vi "信号监控.vi"() -> ()   [LabVIEW 2015]
uses:
  Global control/global-1.vi
  Global control/global-opc.vi
  <userlib>/QMH/Message Queue/Support/Enqueue Message (Single).vi
  Global control/global-2.vi
  <userlib>/QMH/User Event - Stop/User Event - Stop.lvlib
  <userlib>/QMH/Message Queue/Message Queue.lvlib
panel:
  in  "切换界面":bool
  in  "HostThread":variant
  in  "Exit":bool
  in  "选项卡控件":enum32{"继保信号", "管理机信号", "柜体信号"}(tab)
  in  "直流屏-遥测":bool
  in  "直流屏-遥信":bool
  in  "继保选项卡":enum32{"继遥信", "继遥测", "继遥控"}(tab)
  out "继保遥信":T1
  out "继保遥测":T2
  in  "继保遥控":cluster{"断路器分闸":bool, "断路器合闸":bool}
  in  "管理机选项卡":enum32{"管遥信", "管遥测"}(tab)
  out "管理机遥信":T3
  out "管理机遥测":T4 {"主机交流输入电压C相" format="%1.1f"; "主机交流输入电压B相" format="%1.1f"; "主机交流输入电压A相" format="%1.1f"; "母线对地交流电压" format="%1.1f"; "母线负对地电阻" format="%1.1f"; "母线正对地电阻" format="%1.1f"; "母线负对地电压" format="%1.1f"; "母线正对地电压" format="%1.1f"; "负载电流" format="%1.1f"; "母线电压" format="%1.1f"; "电池组温度" format="%1.1f"; "电池组电流" format="%1.1f"; "电池组电压" format="%1.1f"}
  in  "PLC选项卡":T5(tab)
  out "PLC-整流器柜遥测":T6 {"10KV电压输入" format="%1.1f"; "直流1500V电压输出" format="%1.1f"; "直流电流输出" format="%1.1f"}
  in  "PLC-整流器柜遥控":cluster{"模拟中压合闸控制":bool}
  out "PLC-整流器柜遥信":T7
  in  "PLC-直流进线柜遥控":T8
  out "PLC-直流进线柜遥信":T9
  out "PLC-直流馈线柜遥测":cluster{"DC1500V电压输出":dbl} {"DC1500V电压输出" format="%1.1f"}
  in  "PLC-直流馈线柜遥控":T10
  out "PLC-直流馈线柜遥信":T11
  in  "PLC-负极柜遥信遥控":T12
  out "PLC-负极柜遥信":T13
  in  "PLC-接触网隔离开关柜遥控":cluster{"刀开关合闸控制":bool, "刀开关分闸控制":bool}
  out "PLC-接触网隔离开关柜遥信":T14
  # "继保监控"
  # "遥信"
  # "软压板"
  # "开入"
  # "遥测"
  # "遥控"
  # "管理机监控"
  # "遥信"
  # "遥测"
  # "柜体监控"
  # "遥测"
  # "遥控"
  # "遥信"
  # "遥控"
  # "遥信"
  # "遥测"
  # "遥控"
  # "遥信"
  # "遥控"
  # "遥信"
  # "遥控"
  # "遥信"
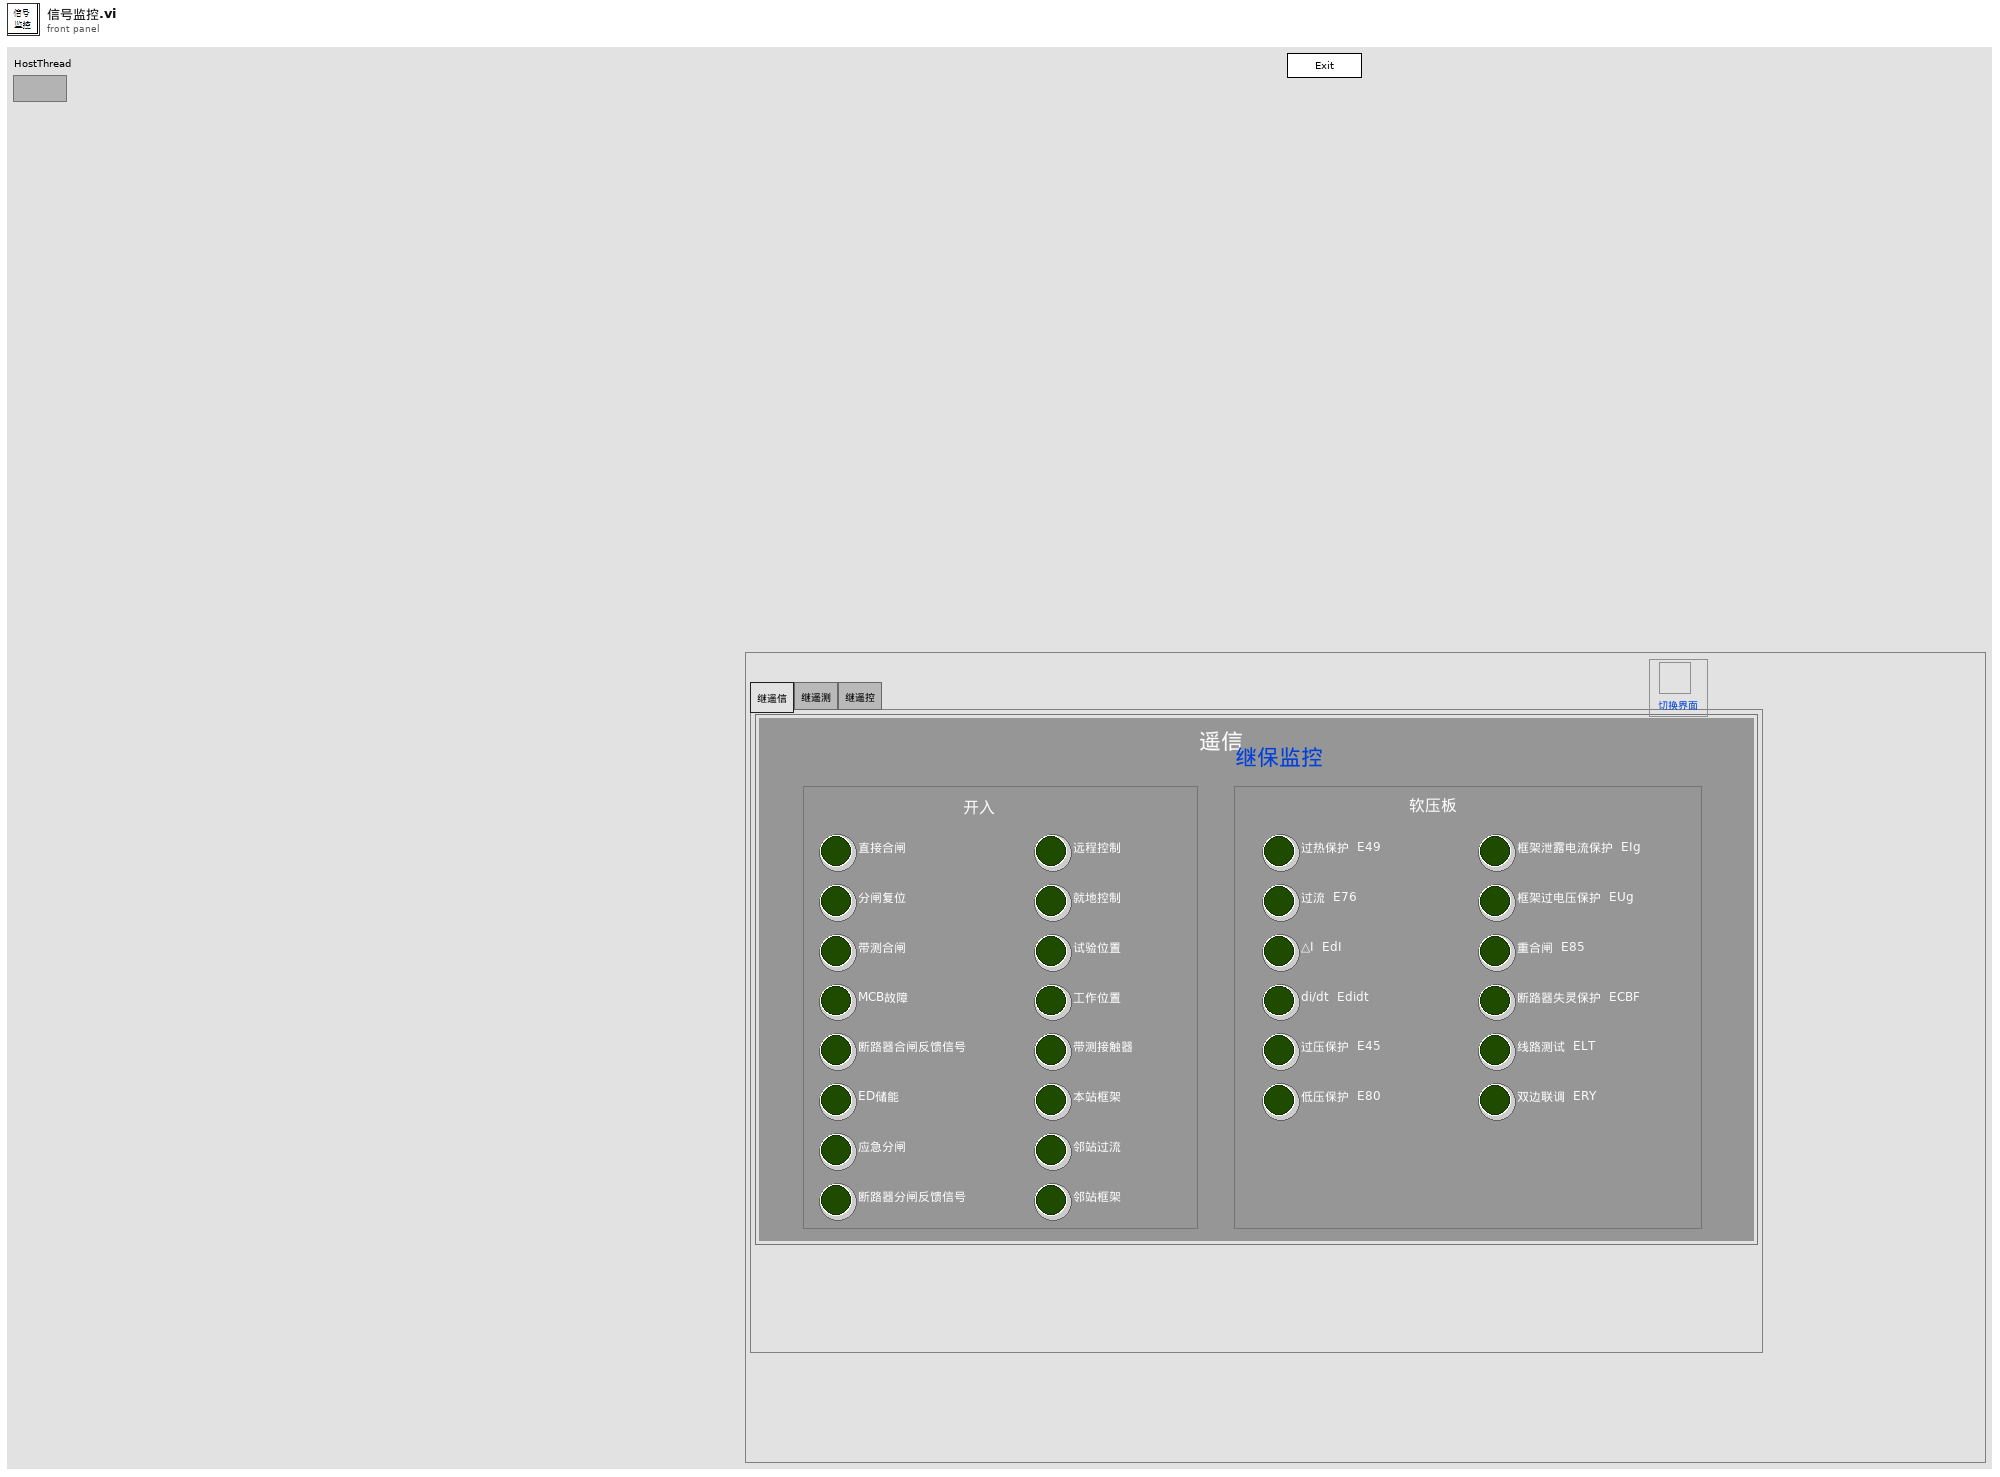
[diagram p1: front panel]
types:
  T1 = cluster{"直接合闸":bool, "分闸复位":bool, "带测合闸":bool, "MCB故障":bool, "断路器合闸反馈信号":bool, "ED储能":bool, "应急分闸":bool, "断路器分闸反馈信号":bool, "远程控制":bool, "就地控制":bool, "试验位置":bool, "工作位置":bool, "带测接触器":bool, "本站框架":bool, "邻站过流":bool, "邻站框架":bool, "过热保护  E49":bool, "过流  E76":bool, "△I  EdI":bool, "di/dt  Edidt":bool, "过压保护  E45":bool, "低压保护  E80":bool, "框架泄露电流保护  EIg":bool, "框架过电压保护  EUg":bool, "重合闸  E85":bool, "断路器失灵保护  ECBF":bool, "线路测试  ELT":bool, "双边联调  ERY":bool}
  T2 = cluster{"电流（I）":u32, "电压（U）":u32, "功率（W）":u32, "框架电流（Ig）":u32, "框架电压（UgV）":u32, "过热余量(Tem)":u32, "电流上升率（didt）":u32, "线路测试状态（LTState）":u32, "重合闸状态（RCLState）":u32}
  T3 = cluster{"母线过压":bool, "母线欠压":bool, "母线绝缘异常":bool, "母线绝缘预警":bool, "母线绝缘压差故障":bool, "母线交流串入故障":bool, "电池组过压":bool, "电池组欠压":bool, "电池组过温":bool, "单体电池故障":bool, "Host交流故障":bool, "Host交流缺相":bool, "Host交流失电":bool, "01#JLCL交流故障":bool, "01#JLCL交流缺相":bool, "01#JLCL交流失电":bool, "02#JLCL交流故障":bool, "02#JLCL交流缺相":bool, "02#JLCL交流失电":bool, "01#电源模块故障":bool, "02#电源模块故障":bool, "03#电源模块故障":bool, "01#模块通信故障":bool, "02#模块通信故障":bool, "03#模块通信故障":bool, "控母输出1#告警":bool, "控母输出2#告警":bool, "控母输出3#告警":bool, "控母输出4#告警":bool, "控母输出5#告警":bool, "控母输出6#告警":bool, "合母输出1#告警":bool, "合母输出2#告警":bool, "合母输出3#告警":bool, "合母输出4#告警":bool, "合母输出5#告警":bool, "合母输出6#告警":bool, "交流输入I告警":bool, "交流输入II告警":bool}
  T4 = cluster{"电池组电压":dbl, "电池组电流":dbl, "电池组温度":dbl, "母线电压":dbl, "负载电流":dbl, "母线正对地电压":dbl, "母线负对地电压":dbl, "母线正对地电阻":dbl, "母线负对地电阻":dbl, "母线对地交流电压":dbl, "主机交流输入电压A相":dbl, "主机交流输入电压B相":dbl, "主机交流输入电压C相":dbl}
  T5 = enum32{"整流器柜", "直流进线柜", "直流馈线柜", "负极柜", "接触网隔离开关柜"}
  T6 = cluster{"直流电流输出":dbl, "直流1500V电压输出":dbl, "10KV电压输入":dbl}
  T7 = cluster{"正常运行":bool, "异常跳闸":bool, "远方":bool, "负极柜故障":bool, "正极柜故障":bool, "馈线柜故障":bool, "接触网隔离开关柜故障":bool, "整流柜跳闸":bool, "整流柜合闸":bool, "压敏快熔故障":bool, "整流柜故障":bool, "模拟中压合闸":bool, "本地":bool}
  T8 = cluster{"刀开关合闸控制":bool, "刀开关分闸控制":bool, "故障复位控制":bool}
  T9 = cluster{"正常运行":bool, "设备准备好":bool, "设备异常":bool, "刀开关合闸完成":bool, "刀开关分闸完成":bool, "刀开关合闸":bool, "刀开关分闸":bool, "复位":bool, "远方":bool, "本地":bool, "刀开关合闸进行中":bool, "刀开关分闸进行中":bool}
  T10 = cluster{"高断储能控制":bool, "旁路合闸控制":bool, "旁路分闸控制":bool, "断路器分闸":bool, "断路器合闸":bool}
  T11 = cluster{"正常运行":bool, "设备准备好":bool, "设备异常":bool, "高断合闸完成":bool, "高断分闸完成":bool, "旁路合闸":bool, "旁路分闸":bool, "继保故障信号":bool, "远方":bool, "本地":bool, "旁路合闸完成":bool, "允许高断合闸":bool}
  T12 = cluster{"模拟框架电流故障控制":bool, "模拟框架电压故障控制":bool, "模拟I段电压故障":bool, "模拟II段电压故障":bool, "故障复位控制":bool}
  T13 = cluster{"正常运行":bool, "设备准备好":bool, "设备异常":bool, "II段电压故障":bool, "MCB故障":bool, "刀开关合闸完成":bool, "复位":bool, "远方":bool, "本地":bool, "装置故障":bool, "刀开关合闸进行中":bool, "框架电流故障":bool, "I段电压故障":bool, "框架电压故障":bool, "刀开关分闸完成":bool}
  T14 = cluster{"正常运行":bool, "设备准备好":bool, "设备异常":bool, "刀开关合闸完成":bool, "刀开关分闸完成":bool, "接触轨有压":bool, "远方":bool, "本地":bool, "刀开关分闸进行中":bool, "刀开关合闸进行中":bool, "刀开关分闸":bool, "刀开关合闸":bool}
  T15 = cluster{"Controls":cluster{"Exit":refnum<vi>}, "Thread":cluster{"ThisQ":string, "ThisVI":refnum<vi>, "HostQ":string, "HostRef":refnum<vi>, "SlavesQ":string[], "SlavesRef":refnum<vi>[]}, "Data":cluster{"Replace":bool}, "User":cluster{"Name":string}}
  T16 = cluster{"高断储能控制":bool, "旁路合闸控制":bool, "旁路分闸控制":bool, "旁路分闸控制 2":bool, "旁路合闸控制 2":bool}
  T17 = cluster{"直接合闸":bool, "分闸复位":bool, "带测合闸":bool, "MCB故障":bool, "断路器合闸反馈信号":bool, "ED储能":bool, "应急分闸":bool, "断路器分闸反馈信号":bool, "远程控制":bool, "就地控制":bool, "试验位置":bool, "工作位置":bool, "带测接触器":bool, "本站框架":bool, "邻站过流":bool, "邻站框架":bool}
  T18 = cluster{"过热保护  E49":bool, "过流  E76":bool, "△I  EdI":bool, "di/dt  Edidt":bool, "过压保护  E45":bool, "低压保护  E80":bool, "框架泄露电流保护  EIg":bool, "框架过电压保护  EUg":bool, "重合闸  E85":bool, "断路器失灵保护  ECBF":bool, "线路测试  ELT":bool, "双边联调  ERY":bool}
  T19 = cluster{"toHMI正常运行":bool, "toHMI异常跳闸":bool, "toHMI远程":bool, "toHMI模拟中压合闸—按钮":bool, "toHMI负极柜故障报警":bool, "toHMI正极柜故障报警":bool, "toHMI馈线柜故障报警":bool, "toHMI上网柜故障报警":bool, "toHMI整流柜故障报警":bool, "toHMI压敏快熔故障":bool, "toHMI整流柜跳闸":bool, "toHMI整流柜合闸—状态":bool, "直流电流输出":u32, "直流220V电压输出":u32, "380电压输入":u32, "模拟中压合闸控制":bool, "toHMI本地":bool}
  T20 = cluster{"toHMI正常运行":bool, "toHMI设备准备好":bool, "toHMI设备异常":bool, "toHMI刀开关合—状态":bool, "toHMI刀开关分—状态":bool, "toHMI刀开关合按钮":bool, "toHMI刀开关分按钮":bool, "toHMI复位按钮":bool, "toHMI远程":bool, "toHMI本地":bool, "toHMI刀闸合—动作":bool, "toHMI刀闸分—动作":bool, "刀开关合闸控制":bool, "刀开关分闸控制":bool, "故障复位控制":bool}
  T21 = cluster{"toHMI正常运行":bool, "toHMI设备准备好":bool, "toHMI设备异常":bool, "toHMI高断分—状态":bool, "toHMI高断合—状态":bool, "toHMI继保故障信号":bool, "toHMI远方":bool, "toHMI本地":bool, "toHMI旁路合闸—按钮":bool, "toHMI旁路分闸—按钮":bool, "toHMI允许高断合闸—状态":bool, "toHMI旁路合分闸—状态":bool, "1500V电压输出":u32, "高断储能控制":bool, "旁路合闸控制":bool, "旁路分闸控制":bool}
  T22 = cluster{"toHMI正常运行":bool, "toHMI设备准备好":bool, "toHMI设备异常":bool, "toHMI刀开关分—状态":bool, "toHMI刀开关合—状态":bool, "toHMI框架电流故障":bool, "toHMI框架电压故障":bool, "toHMII段电压故障":bool, "toHMIII段电压故障":bool, "toHMI装置故障":bool, "toHMIMCB故障":bool, "toHMI刀开关合—完成":bool, "toHMI复位按钮":bool, "toHMI远程":bool, "toHMI本地":bool, "模拟电流框架故障控制":bool, "模拟电压框架故障控制":bool, "模拟I段电压故障控制":bool, "模拟II段电压故障控制":bool, "故障复位控制":bool}
  T23 = cluster{"toHMI刀开关合—状态":bool, "toHMI刀开关分—状态":bool, "toHMI刀开关合按钮":bool, "toHMI刀开关分按钮":bool, "toHMI远程":bool, "toHMI本地":bool, "toHMI正常运行":bool, "toHMI设备准备好":bool, "toHMI设备异常":bool, "toHMI刀闸合—动作":bool, "toHMI刀闸分—动作":bool, "toHMI接触轨有压":bool, "刀开关合闸控制":bool, "刀开关分闸控制":bool}
  T24 = cluster{"母线过压":bool, "母线欠压":bool, "母线绝缘异常":bool, "母线绝缘预警":bool, "母线绝缘压差故障":bool, "母线交流串入故障":bool, "备用5":bool, " 备用6":bool, "电池组过压":bool, "电池组欠压":bool, "电池组过温":bool, "单体电池故障":bool, "备用1":bool, "备用2":bool, "备用3":bool, " 备用4":bool}
  T25 = cluster{"Host交流故障":bool, "Host交流缺相":bool, "Host交流失电":bool, "01#JLCL交流故障":bool, "01#JLCL交流缺相":bool, "01#JLCL交流失电":bool, "02#JLCL交流故障":bool, "02#JLCL交流缺相":bool, "02#JLCL交流失电":bool, "备用1":bool, "备用2":bool, "备用3":bool, "备用4":bool, "备用5":bool, "备用6":bool, " 备用7":bool}
  T26 = cluster{"09#电源模块故障":bool, "10#电源模块故障":bool, "11#电源模块故障":bool, "12#电源模块故障":bool, "13#电源模块故障":bool, "14#电源模块故障":bool, "15#电源模块故障":bool, "16#电源模块故障":bool, "01#电源模块故障":bool, "02#电源模块故障":bool, "03#电源模块故障":bool, "04#电源模块故障":bool, "05#电源模块故障":bool, "06#电源模块故障":bool, "07#电源模块故障":bool, " 08#电源模块故障":bool}
  T27 = cluster{"09#模块通信故障":bool, "10#模块通信故障":bool, "11#模块通信故障":bool, "12#模块通信故障":bool, "13#模块通信故障":bool, "14#模块通信故障":bool, "15#模块通信故障":bool, "16#模块通信故障":bool, "01#模块通信故障":bool, "02#模块通信故障":bool, "03#模块通信故障":bool, "04#模块通信故障":bool, "05#模块通信故障":bool, "06#模块通信故障":bool, "07#模块通信故障":bool, "08#模块通信故障":bool}
  T28 = cluster{"25#开关状态":bool, "26#开关状态":bool, "27#开关状态":bool, "28#开关状态":bool, "29#开关状态":bool, "30#开关状态":bool, "31#开关状态":bool, "32#开关状态":bool, "交流输入I告警":bool, "交流输入II告警":bool, "19#开关状态":bool, "20#开关状态":bool, "21#开关状态":bool, "22#开关状态":bool, "23#开关状态":bool, "24#开关状态":bool}
  T29 = cluster{"合母输出3#告警":bool, "合母输出4#告警":bool, "合母输出5#告警":bool, "合母输出6#告警":bool, "13#开关状态":bool, "14#开关状态":bool, "15#开关状态":bool, "16#开关状态":bool, "控母输出1#告警":bool, "控母输出2#告警":bool, "控母输出3#告警":bool, "控母输出4#告警":bool, "控母输出5#告警":bool, "控母输出6#告警":bool, "合母输出1#告警":bool, "合母输出2#告警":bool}
  T30 = cluster{"直流电流输出":u32, "直流220V电压输出":u32, "380电压输入":u32}
  T31 = cluster{"整流柜远程/本地":enum16{"零位", "本地", "远方"}, "进线柜远程/本地":enum16{"零位", "本地", "远方"}, "馈线柜远程/本地":enum16{"零位", "本地", "远方"}, "负极柜远程/本地":enum16{"零位", "本地", "远方"}, "上网柜远程/本地":enum16{"零位", "本地", "远方"}, "直流继保远程/本地":enum16{"零位", "本地", "远方"}}
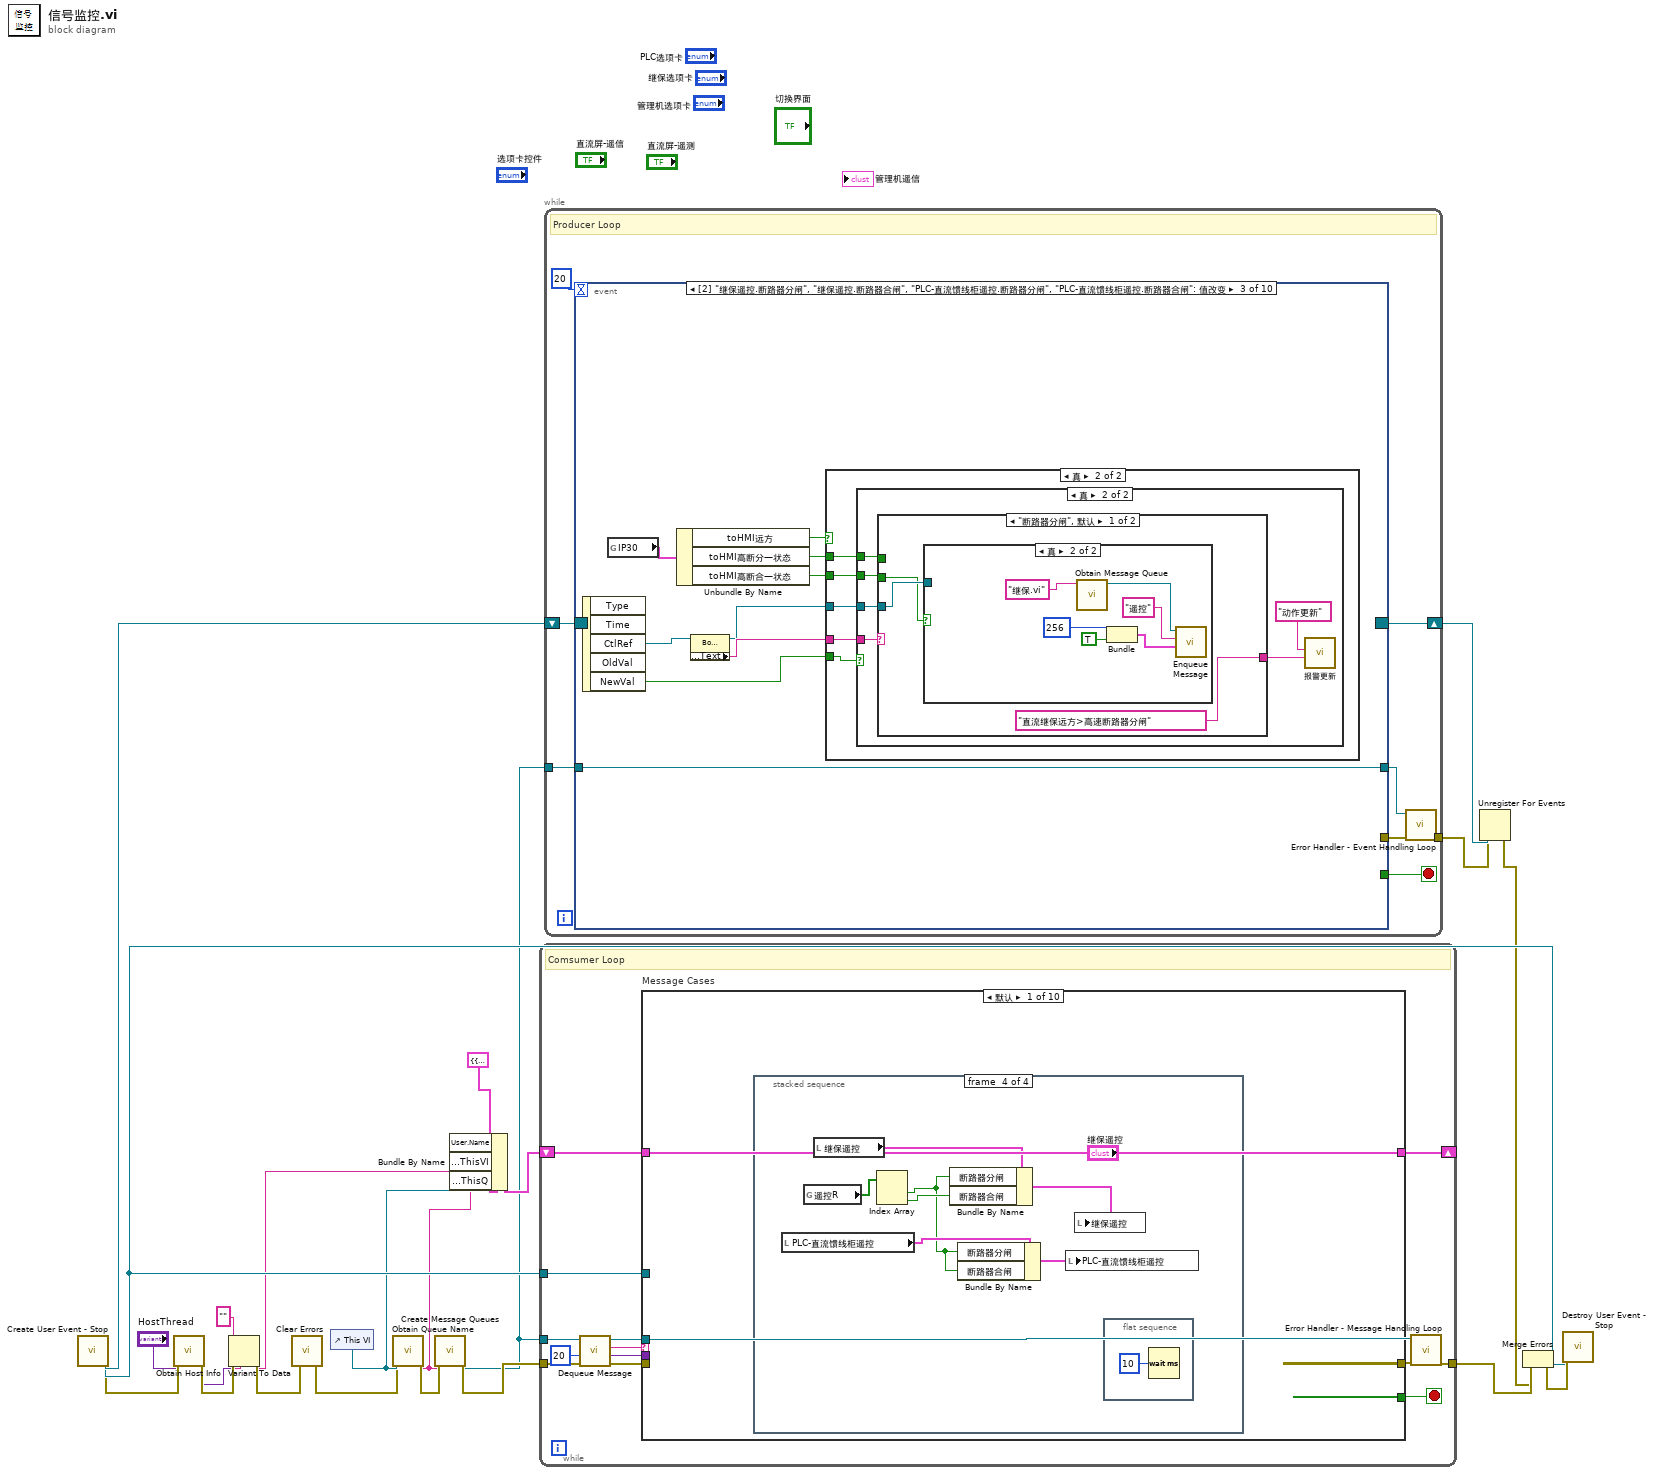
[diagram p0: block diagram]
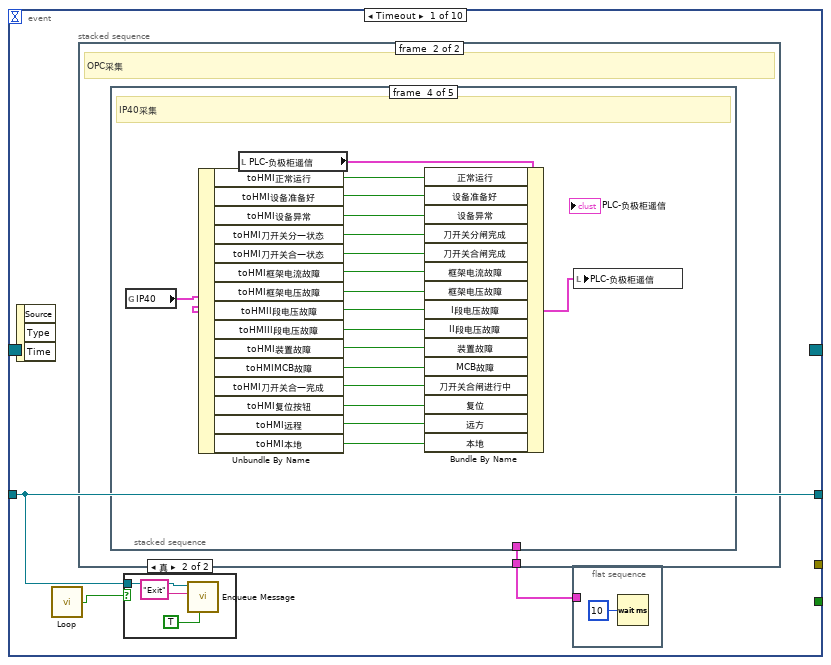
[diagram p2: hidden frame]
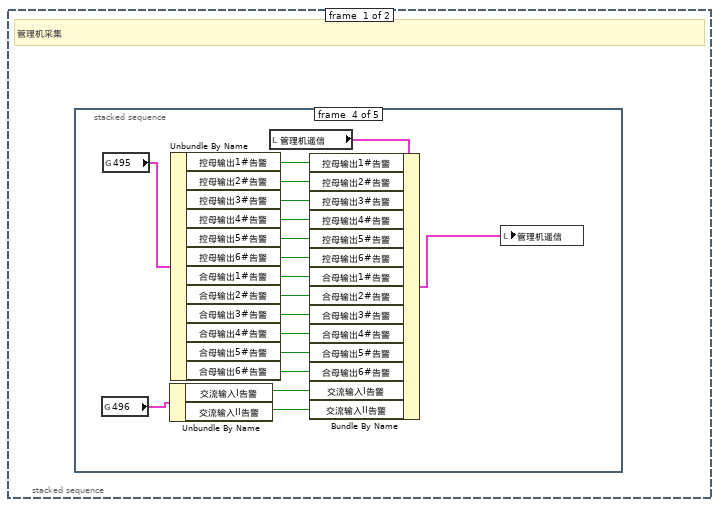
[diagram p3: hidden frame]
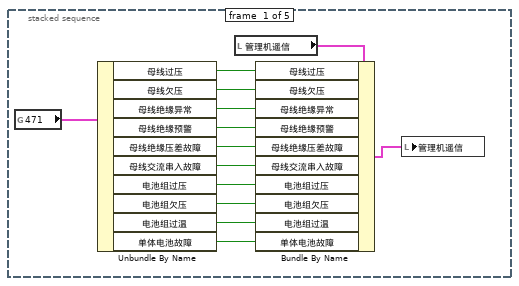
[diagram p4: hidden frame]
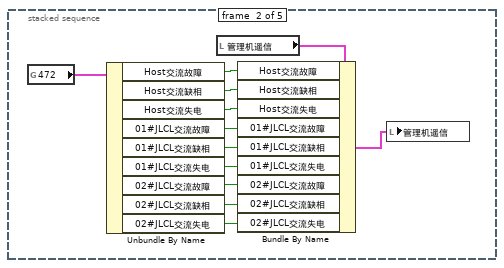
[diagram p5: hidden frame]
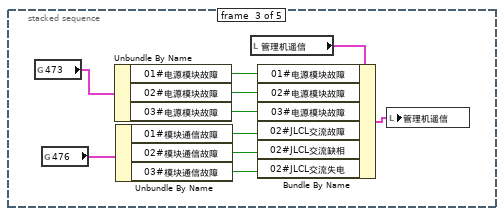
[diagram p6: hidden frame]
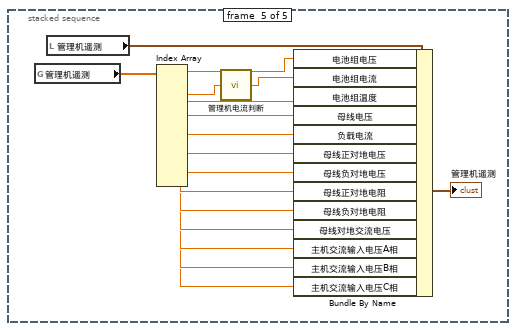
[diagram p7: hidden frame]
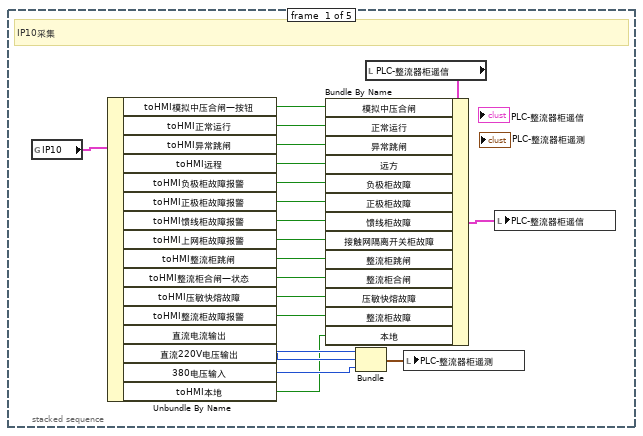
[diagram p8: hidden frame]
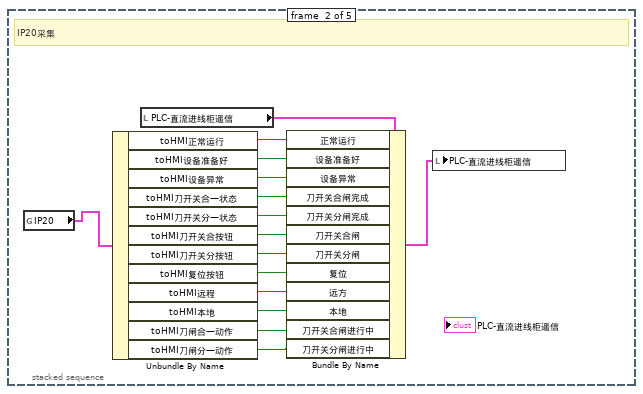
[diagram p9: hidden frame]
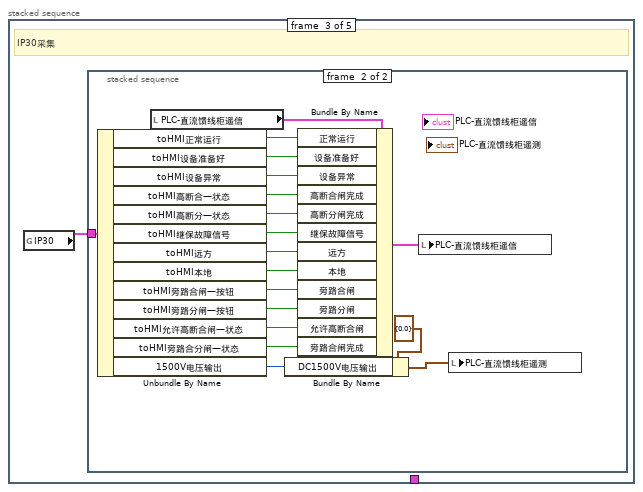
[diagram p10: hidden frame]
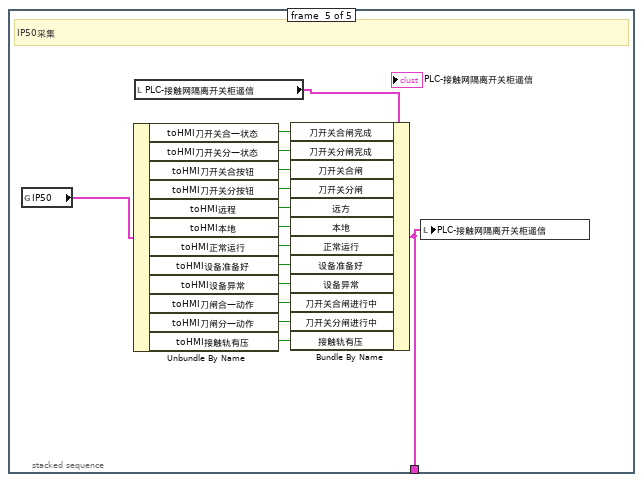
[diagram p12: hidden frame]
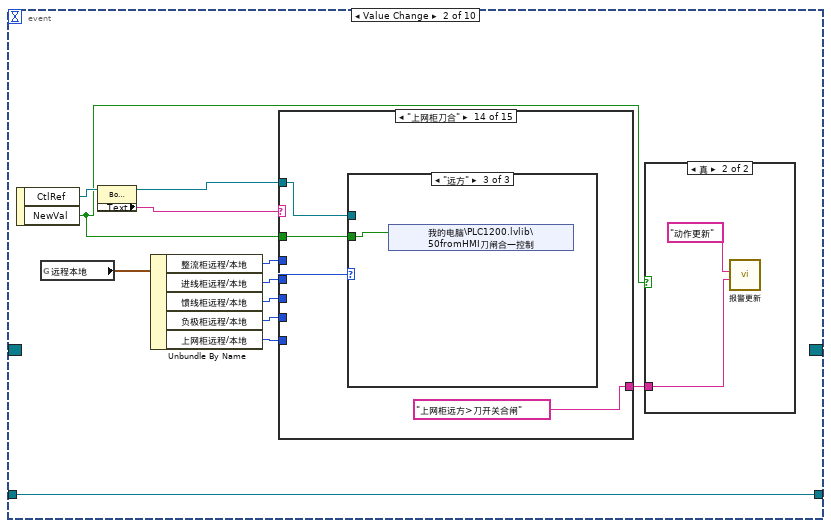
[diagram p14: hidden frame]
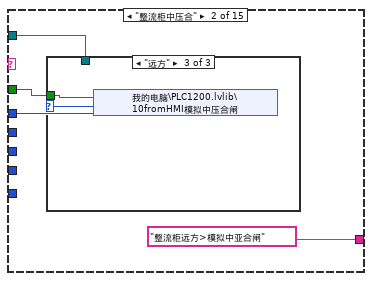
[diagram p17: hidden frame]
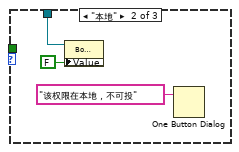
[diagram p19: hidden frame]
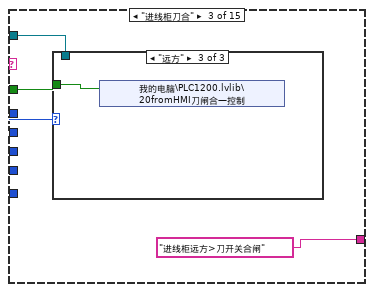
[diagram p20: hidden frame]
diagram:
  n1 = call <userlib>:"Create User Event - Stop.vi"() -> ("error out"=w9:errorcluster, "User Event - Stop"=w18:refnum<user-event>, "Stop Event Registration Refnum"=w20:refnum<event-registration>)  [unwired: 9 in]
  n2 = call <userlib>:"Obtain Host Info.vi"("error in (no error)"=w9, "HostThread"="HostThread") -> ("error out"=w6:errorcluster, "Data"=w5:variant)  [unwired: 6 in, 2 out]
  n3 = Variant To Data(error in=w6, type="", Variant=w5) -> (data=w1:string, error out=w3:errorcluster)
  n4 = call <vilib>:"Clear Errors.vi"("error in (no error)"=w3) -> ("error out"=w2:errorcluster)  [unwired: 5 in, 1 out]
  n5 = control-ref of="This VI"() -> (w11:refnum<vi>)
  n6 = call <userlib>:"Obtain Queue Name.vi"("error in (no error)"=w2, "VI Refnum"=w11) -> ("error out"=w14:errorcluster, "ViName"=w10:string)  [unwired: 8 in]
  n7 = call <userlib>:"Create Message Queues.vi"("error in (no error)"=w14, "name (unnamed)"=w10) -> ("error out"=w22:errorcluster, "QueueHandler"=w7:refnum<queue>)  [unwired: 8 in]
  n8 = Bundle By Name(cluster=T15 {"Controls"={"Exit"=refnum}, "Thread"={"ThisQ"="", "ThisVI"=refnum, "HostQ"="", "HostRef"=refnum, "SlavesQ"=[], "SlavesRef"=[]}, "Data"={"Replace"=FALSE}, "User"={"Name"=""}} ("Data Cluster"), "User.Name"=w1, "Thread.ThisVI"=w11, "Thread.ThisQ"=w10) -> (w12:T15)
  n9 = while {
    tunnel: w7 -> [w27]
    shift-right: [w34] -> _
    shift-left: w12 -> [w35]
    tunnel: w18 -> [w32]
    tunnel: w22 -> [w31]
    tunnel: [w25] -> w21
    stop <- w33 stop-if-true
    # "Comsumer Loop"
    n10 = call <userlib>:"Dequeue Message.vi"("error in (no error)"=w31, "timeout in ms (-1)"=20, "Message Queue"=w27) -> ("error out"=w30:errorcluster, "Message Data"=w28:variant, "Message"=w29:string, "dup Message Queue"=w26:refnum<queue>)  [unwired: 5 in]
    n11 = case "Message Cases" shown="默认" w29 {
      tunnel: w26 -> [_ w98 _ w115 _ _ _ _ _ _]
      tunnel: w30 -> [_ w93 w112 w119 w125 w171 w173 w175 w176 w179]
      tunnel: [_ w94 w107 w117 w125 w171 w173 w175 w176 w179] -> w24
      tunnel: w35 -> [w36 w97 w104 w118 w126 w170 w172 w174 w177 w178]
      tunnel: [w36 w97 w104 w118 w126 w170 w172 w174 w177 w178] -> w34
      tunnel: [_ TRUE _ _ _ _ _ _ _ _] -> w33
      tunnel: w28 -> [_ _ w111 _ _ _ _ _ _ _]
      tunnel: w32 -> [_ w92 _ _ _ _ _ _ _ _]
      frame Default {
        # "'Default' case only runs if there is a message that isn't defined in any of the other cases.  Output a programming error."
        n12 = stacked-sequence {
          frame #0 {
            n13 = global read "global-2.vi" "开入"() -> (w53:T17)
            n14 = local read "继保遥信"() -> (w55:T1)
            n15 = Unbundle By Name(w53) -> ("直接合闸"=w52:bool, "分闸复位"=w51:bool, "带测合闸"=w50:bool, "MCB故障"=w49:bool, "断路器合闸反馈信号"=w48:bool, "ED储能"=w47:bool, "应急分闸"=w46:bool, "断路器分闸反馈信号"=w45:bool, "远程控制"=w44:bool, "就地控制"=w43:bool, "试验位置"=w42:bool, "工作位置"=w41:bool, "带测接触器"=w40:bool, "本站框架"=w39:bool, "邻站过流"=w38:bool, "邻站框架"=w37:bool)
            n16 = Bundle By Name(cluster=w55, "直接合闸"=w52, "分闸复位"=w51, "带测合闸"=w50, "MCB故障"=w49, "断路器合闸反馈信号"=w48, "ED储能"=w47, "应急分闸"=w46, "断路器分闸反馈信号"=w45, "远程控制"=w44, "就地控制"=w43, "试验位置"=w42, "工作位置"=w41, "带测接触器"=w40, "本站框架"=w39, "邻站过流"=w38, "邻站框架"=w37) -> (→"继保遥信":T1)
          }
          frame #1 {
            n17 = local read "继保遥信"() -> (w70:T1)
            n18 = global read "global-2.vi" "软压板R"() -> (w68:T18)
            n19 = Unbundle By Name(w68) -> ("过热保护  E49"=w67:bool, "过流  E76"=w66:bool, "△I  EdI"=w65:bool, "di/dt  Edidt"=w64:bool, "过压保护  E45"=w63:bool, "低压保护  E80"=w62:bool, "框架泄露电流保护  EIg"=w61:bool, "框架过电压保护  EUg"=w60:bool, "重合闸  E85"=w59:bool, "断路器失灵保护  ECBF"=w58:bool, "线路测试  ELT"=w57:bool, "双边联调  ERY"=w56:bool)
            n20 = Bundle By Name(cluster=w70, "过热保护  E49"=w67, "过流  E76"=w66, "△I  EdI"=w65, "di/dt  Edidt"=w64, "过压保护  E45"=w63, "低压保护  E80"=w62, "框架泄露电流保护  EIg"=w61, "框架过电压保护  EUg"=w60, "重合闸  E85"=w59, "断路器失灵保护  ECBF"=w58, "线路测试  ELT"=w57, "双边联调  ERY"=w56) -> (w69:T1)
            n21 = local write "继保遥信"(w69) -> ()
          }
          frame #2 {
            n22 = local read "继保遥测"() -> (w82:T2)
            n23 = global read "global-2.vi" "遥测"() -> (w81:u32[])
            n24 = Index Array(array=w81) -> (element #1=w80:u32, element #2=w79:u32, element #3=w78:u32, element #4=w77:u32, element #5=w76:u32, element #6=w75:u32, element #7=w74:u32, element #8=w73:u32, element #9=w72:u32)  [unwired: 9 in]
            n25 = Bundle By Name(cluster=w82, "电流（I）"=w80, "电压（U）"=w79, "功率（W）"=w78, "框架电流（Ig）"=w77, "框架电压（UgV）"=w76, "过热余量(Tem)"=w75, "电流上升率（didt）"=w74, "线路测试状态（LTState）"=w73, "重合闸状态（RCLState）"=w72) -> (→"继保遥测":T2)
          }
          frame #3 {
            n26 = local read "PLC-直流馈线柜遥控"() -> (w85:T10)
            n27 = global read "global-2.vi" "遥控R"() -> (w88:bool[])
            n28 = local read "继保遥控"() -> (w89:cluster{"断路器分闸":bool, "断路器合闸":bool})
            n29 = Index Array(array=w88) -> (element #1=w83:bool, element #2=w87:bool)  [unwired: 2 in]
            n30 = Bundle By Name(cluster=w89, "断路器分闸"=w83, "断路器合闸"=w87) -> (w86:cluster{"断路器分闸":bool, "断路器合闸":bool})
            n31 = Bundle By Name(cluster=w85, "断路器分闸"=w83, "断路器合闸"=w83) -> (w84:T10)
            n32 = local write "PLC-直流馈线柜遥控"(w84) -> ()
            n33 = local write "继保遥控"(w86) -> ()
            n34 = flat-sequence {
              frame #0 {
                n35 = Wait (ms)(milliseconds to wait=u32 10 ("等待时间（毫秒）")) -> ()  [unwired: 1 out]
              }
            }
          }
        }
      }
      frame "Exit" {
        # "Stop the VI"
        # "Release the message queue reference"
        # "#CodeNeeded - Add any required cleanup code here"
        # "Exit - Exit the application."
        n36 = call <userlib>:"Fire User Event - Stop.vi"("User Event - Stop"=w92) -> ("error out"=w91:errorcluster)  [unwired: 10 in]
        n37 = Release Queue(queue=w98, error in (no error)=w93) -> (error out=w95:errorcluster)  [unwired: 1 in, 2 out]
        n38 = Merge Errors(w91, w95) -> (w94:errorcluster)
      }
      frame "Error" {
        # "Error - Check the error message data and respond accordingly. This message is sent by the \"Error Handler\" VIs at the end of each loop in this application."
        n39 = Unbundle By Name(w104) -> ("Thread.HostQ"=w103:string)
        n40 = Variant To Data(error in=w112, type=errorcluster {"status"=FALSE, "code"=0, "source"=""} ("error constant"), Variant=w111) -> (data=w100:errorcluster, error out=w109:errorcluster)
        n41 = To Variant(anything=w100) -> (Variant=w99:variant)
        n42 = call <userlib>:"Obtain Message Queue.vi"("name (unnamed)"=w103) -> ("error out"=w102:errorcluster, "Message Queue"=w101:refnum<queue>)  [unwired: 9 in]
        n43 = call-poly <userlib>:"Enqueue Message.vi"("Priority Message? (F)"=TRUE, "error in (no error)"=w102, "Message Data"=w99, "Message"="Error", "Message Queue"=w101) -> ("error out"=w108:errorcluster)  [unwired: 5 in, 1 out]
        n44 = Merge Errors(w108, w109) -> (w107:errorcluster)
      }
      frame "Confirm Quit" {
        # "#CodeNeeded - If you want to provide an \"Are you sure\" dialog (or some other notification) before the application exits, place that code here. This message is typically sent from a Panel Close? event."
        # "Confirm Quit - Message that can confirm whether or not the user wants to exit the application."
        n45 = call-poly <userlib>:"Enqueue Message.vi"("Priority Message? (F)"=TRUE, "error in (no error)"=w119, "Message"="Exit", "Message Queue"=w115) -> ("error out"=w116:errorcluster)  [unwired: 6 in, 1 out]
        n46 = Merge Errors(w116) -> (w117:errorcluster)
      }
      frame "Initialize" {
        # "Initialize - Send separate messages to initialize the data and the front panel.  Bundle control references."
        n47 = local write "PLC-接触网隔离开关柜遥控"(cluster{"刀开关合闸控制":bool, "刀开关分闸控制":bool} {"刀开关合闸控制"=FALSE, "刀开关分闸控制"=FALSE} ("PLC-接触网隔离开关柜遥控")) -> ()
        n48 = local write "PLC-负极柜遥信遥控"(T12 {"模拟框架电流故障控制"=FALSE, "模拟框架电压故障控制"=FALSE, "模拟I段电压故障"=FALSE, "模拟II段电压故障"=FALSE, "故障复位控制"=FALSE} ("PLC-负极柜遥信遥控")) -> ()
        n49 = stacked-sequence {
          frame #0 {
            n50 = shared-variable "我的电脑\\PLC1200.lvlib\\50fromHMI刀闸合—控制"(FALSE) -> ()  [unwired: 1 in, 1 out]
            n51 = shared-variable "我的电脑\\PLC1200.lvlib\\40fromHMI模拟框架电压故障"(FALSE) -> ()  [unwired: 1 in, 1 out]
            n52 = shared-variable "我的电脑\\PLC1200.lvlib\\50fromHMI刀闸分—控制"(FALSE) -> ()  [unwired: 1 in, 1 out]
            n53 = shared-variable "我的电脑\\PLC1200.lvlib\\40fromHMI模拟框架电流故障"(FALSE) -> ()  [unwired: 1 in, 1 out]
            n54 = shared-variable "我的电脑\\PLC1200.lvlib\\40fromHMI模拟I段电压故障"(FALSE) -> ()  [unwired: 1 in, 1 out]
            n55 = shared-variable "我的电脑\\PLC1200.lvlib\\40fromHMI模拟II段电压故障"(FALSE) -> ()  [unwired: 1 in, 1 out]
            n56 = shared-variable "我的电脑\\PLC1200.lvlib\\40fromHMI故障复位"(FALSE) -> ()  [unwired: 1 in, 1 out]
            n57 = shared-variable "我的电脑\\PLC1200.lvlib\\30fromHMI旁路分闸—控制"(FALSE) -> ()  [unwired: 1 in, 1 out]
            n58 = shared-variable "我的电脑\\PLC1200.lvlib\\30fromHMI旁路合闸—控制"(FALSE) -> ()  [unwired: 1 in, 1 out]
            n59 = shared-variable "我的电脑\\PLC1200.lvlib\\30fromHMI高断储能—控制"(FALSE) -> ()  [unwired: 1 in, 1 out]
            n60 = shared-variable "我的电脑\\PLC1200.lvlib\\20fromHMI刀闸分—控制"(FALSE) -> ()  [unwired: 1 in, 1 out]
            n61 = shared-variable "我的电脑\\PLC1200.lvlib\\20fromHMI刀闸合—控制"(FALSE) -> ()  [unwired: 1 in, 1 out]
            n62 = shared-variable "我的电脑\\PLC1200.lvlib\\20fromHMI故障复位"(FALSE) -> ()  [unwired: 1 in, 1 out]
            n63 = shared-variable "我的电脑\\PLC1200.lvlib\\10fromHMI模拟中压合闸"(FALSE) -> ()  [unwired: 1 in, 1 out]
          }
          frame #1 {
            n64 = global read "global-opc.vi" "IP10"() -> (w141:T19)
            n65 = Unbundle By Name(w141) -> ("模拟中压合闸控制"=w143:bool)
            n66 = local read "PLC-整流器柜遥控"() -> (w144:cluster{"模拟中压合闸控制":bool})
            n67 = Bundle By Name(cluster=w144, "模拟中压合闸控制"=w143) -> (w142:cluster{"模拟中压合闸控制":bool})
            n68 = local write "PLC-整流器柜遥控"(w142) -> ()
          }
          frame #2 {
            n69 = global read "global-opc.vi" "IP20"() -> (w145:T20)
            n70 = Unbundle By Name(w145) -> ("刀开关合闸控制"=w148:bool, "刀开关分闸控制"=w149:bool, "故障复位控制"=w150:bool)
            n71 = local read "PLC-直流进线柜遥控"() -> (w146:T8)
            n72 = Bundle By Name(cluster=w146, "刀开关合闸控制"=w148, "刀开关分闸控制"=w149, "故障复位控制"=w150) -> (w147:T8)
            n73 = local write "PLC-直流进线柜遥控"(w147) -> ()
          }
          frame #3 {
            n74 = global read "global-opc.vi" "IP30"() -> (w151:T21)
            n75 = Unbundle By Name(w151) -> ("高断储能控制"=w153:bool, "旁路合闸控制"=w154:bool, "旁路分闸控制"=w155:bool)
            n76 = local read "PLC-直流馈线柜遥控"() -> (w152:T10)
            n77 = Bundle By Name(cluster=w152, "高断储能控制"=w153, "旁路合闸控制"=w154, "旁路分闸控制"=w155) -> (w156:T10)
            n78 = local write "PLC-直流馈线柜遥控"(w156) -> ()
          }
          frame #4 {
            n79 = global read "global-opc.vi" "IP40"() -> (w157:T22)
            n80 = Unbundle By Name(w157) -> ("模拟电流框架故障控制"=w160:bool, "模拟电压框架故障控制"=w161:bool, "模拟I段电压故障控制"=w162:bool, "模拟II段电压故障控制"=w163:bool, "故障复位控制"=w164:bool)
            n81 = local read "PLC-负极柜遥信遥控"() -> (w158:T12)
            n82 = Bundle By Name(cluster=w158, "模拟框架电流故障控制"=w160, "模拟框架电压故障控制"=w161, "模拟I段电压故障"=w162, "模拟II段电压故障"=w163, "故障复位控制"=w164) -> (w159:T12)
            n83 = local write "PLC-负极柜遥信遥控"(w159) -> ()
          }
          frame #5 {
            n84 = global read "global-opc.vi" "IP50"() -> (w165:T23)
            n85 = local read "PLC-接触网隔离开关柜遥控"() -> (w166:cluster{"刀开关合闸控制":bool, "刀开关分闸控制":bool})
            n86 = Unbundle By Name(w165) -> ("刀开关合闸控制"=w167:bool, "刀开关分闸控制"=w168:bool)
            n87 = Bundle By Name(cluster=w166, "刀开关合闸控制"=w167, "刀开关分闸控制"=w168) -> (w169:cluster{"刀开关合闸控制":bool, "刀开关分闸控制":bool})
            n88 = local write "PLC-接触网隔离开关柜遥控"(w169) -> ()
          }
        }
        n89 = local write "PLC-整流器柜遥控"(cluster{"模拟中压合闸控制":bool} {"模拟中压合闸控制"=FALSE} ("PLC-整流器柜遥控")) -> ()
        n90 = local write "PLC-直流进线柜遥控"(T8 {"刀开关合闸控制"=FALSE, "刀开关分闸控制"=FALSE, "故障复位控制"=FALSE} ("PLC-直流进线柜遥控")) -> ()
        n91 = local write "PLC-直流馈线柜遥控"(T16 {"高断储能控制"=FALSE, "旁路合闸控制"=FALSE, "旁路分闸控制"=FALSE, "旁路分闸控制 2"=FALSE, "旁路合闸控制 2"=FALSE} ("PLC-直流馈线柜遥控")) -> ()
      }
      frame "控制" {
      }
      frame "<-------UI-------->" {
      }
      frame "<------Core------>" {
      }
      frame "Core_InitializeRef" {
        # "Initialize control references. For there is not enough space to locate all the control references, separate the codes into 2 messages"
      }
      frame "<---Operation--->" {
      }
    }
    n92 = call <userlib>:"Error Handler - Message Handling Loop.vi"("error in (no error)"=w24, "Message Queue"=w26) -> ("dup error in"=w25:errorcluster)  [unwired: 8 in, 1 out]
  }
  n93 = while {
    tunnel: w7 -> [w187]
    shift-right: [w185] -> w16
    shift-left: w20 -> [w186]
    tunnel: [w181] -> w15
    stop <- w183 stop-if-true
    # "Producer Loop"
    n94 = event shown="[2] \"继保遥控.断路器分闸\", \"继保遥控.断路器合闸\", \"PLC-直流馈线柜遥控.断路器分闸\", \"PLC-直流馈线柜遥控.断路器合闸\": 值改变" {
      selector: w186 -> [_ _ _ _ _ _ _ _ _ _]
      dyn-events: [_ _ _ _ _ _ _ _ _ _] -> w185
      timeout: 20 -> [_ _ _ _ _ _ _ _ _ _]
      tunnel: [_ _ _ _ _ TRUE ("Discard?") _ _ _ _] -> w183
      tunnel: w187 -> [w189 w364 w494 w537 w539 w541 w546 w549 w554 w565]
      tunnel: [_ _ _ w536 _ _ w544 _ _ _] -> w184
      tunnel: [w189 w364 w494 w535 w539 w541 w545 w549 w554 w565] -> w182
      event Timeout {
        # "Add circle collection here; And according to the different signal, we should build the \"Choose Box\"."
        n95 = event-data() -> ()  [unwired: 1 in, 3 out]
        n96 = call "Loop.vi"() -> ("Loop Out"=w190:bool)  [unwired: 5 in]
        n97 = stacked-sequence {
          tunnel: [_ w262] -> w188
          frame #0 {
            # "管理机采集"
            n98 = stacked-sequence {
              frame #0 {
                n99 = global read "global-1.vi" "471"() -> (w204:T24)
                n100 = Unbundle By Name(w204) -> ("母线过压"=w203:bool, "母线欠压"=w202:bool, "母线绝缘异常"=w201:bool, "母线绝缘预警"=w200:bool, "母线绝缘压差故障"=w199:bool, "母线交流串入故障"=w198:bool, "电池组过压"=w197:bool, "电池组欠压"=w196:bool, "电池组过温"=w195:bool, "单体电池故障"=w194:bool)
                n101 = local read "管理机遥信"() -> (w193:T3)
                n102 = Bundle By Name(cluster=w193, "母线过压"=w203, "母线欠压"=w202, "母线绝缘异常"=w201, "母线绝缘预警"=w200, "母线绝缘压差故障"=w199, "母线交流串入故障"=w198, "电池组过压"=w197, "电池组欠压"=w196, "电池组过温"=w195, "单体电池故障"=w194) -> (w192:T3)
                n103 = local write "管理机遥信"(w192) -> ()
              }
              frame #1 {
                n104 = global read "global-1.vi" "472"() -> (w216:T25)
                n105 = Unbundle By Name(w216) -> ("Host交流故障"=w215:bool, "Host交流缺相"=w214:bool, "Host交流失电"=w213:bool, "01#JLCL交流故障"=w212:bool, "01#JLCL交流缺相"=w211:bool, "01#JLCL交流失电"=w210:bool, "02#JLCL交流故障"=w207:bool, "02#JLCL交流缺相"=w206:bool, "02#JLCL交流失电"=w205:bool)
                n106 = local read "管理机遥信"() -> (w208:T3)
                n107 = Bundle By Name(cluster=w208, "Host交流故障"=w215, "Host交流缺相"=w214, "Host交流失电"=w213, "01#JLCL交流故障"=w212, "01#JLCL交流缺相"=w211, "01#JLCL交流失电"=w210, "02#JLCL交流故障"=w207, "02#JLCL交流缺相"=w206, "02#JLCL交流失电"=w205) -> (w209:T3)
                n108 = local write "管理机遥信"(w209) -> ()
              }
              frame #2 {
                n109 = global read "global-1.vi" "473"() -> (w226:T26)
                n110 = global read "global-1.vi" "476"() -> (w224:T27)
                n111 = Unbundle By Name(w226) -> ("01#电源模块故障"=w217:bool, "02#电源模块故障"=w218:bool, "03#电源模块故障"=w219:bool)
                n112 = Unbundle By Name(w224) -> ("01#模块通信故障"=w225:bool, "02#模块通信故障"=w223:bool, "03#模块通信故障"=w222:bool)
                n113 = local read "管理机遥信"() -> (w221:T3)
                n114 = Bundle By Name(cluster=w221, "01#电源模块故障"=w217, "02#电源模块故障"=w218, "03#电源模块故障"=w219, "02#JLCL交流故障"=w225, "02#JLCL交流缺相"=w223, "02#JLCL交流失电"=w222) -> (w220:T3)
                n115 = local write "管理机遥信"(w220) -> ()
              }
              frame #3 {
                n116 = global read "global-1.vi" "496"() -> (w241:T28)
                n117 = global read "global-1.vi" "495"() -> (w244:T29)
                n118 = Unbundle By Name(w241) -> ("交流输入I告警"=w228:bool, "交流输入II告警"=w227:bool)
                n119 = Unbundle By Name(w244) -> ("控母输出1#告警"=w240:bool, "控母输出2#告警"=w239:bool, "控母输出3#告警"=w238:bool, "控母输出4#告警"=w237:bool, "控母输出5#告警"=w236:bool, "控母输出6#告警"=w235:bool, "合母输出1#告警"=w234:bool, "合母输出2#告警"=w233:bool, "合母输出3#告警"=w232:bool, "合母输出4#告警"=w231:bool, "合母输出5#告警"=w230:bool, "合母输出6#告警"=w229:bool)
                n120 = local read "管理机遥信"() -> (w242:T3)
                n121 = Bundle By Name(cluster=w242, "控母输出1#告警"=w240, "控母输出2#告警"=w239, "控母输出3#告警"=w238, "控母输出4#告警"=w237, "控母输出5#告警"=w236, "控母输出6#告警"=w235, "合母输出1#告警"=w234, "合母输出2#告警"=w233, "合母输出3#告警"=w232, "合母输出4#告警"=w231, "合母输出5#告警"=w230, "合母输出6#告警"=w229, "交流输入I告警"=w228, "交流输入II告警"=w227) -> (w243:T3)
                n122 = local write "管理机遥信"(w243) -> ()
              }
              frame #4 {
                n123 = global read "global-1.vi" "管理机遥测"() -> (w260:dbl[])
                n124 = local read "管理机遥测"() -> (w261:T4)
                n125 = Index Array(array=w260) -> (element #1=w247:dbl, element #2=w246:dbl, element #3=w258:dbl, element #4=w257:dbl, element #5=w256:dbl, element #6=w255:dbl, element #7=w254:dbl, element #8=w253:dbl, element #9=w252:dbl, element #10=w251:dbl, element #11=w250:dbl, element #12=w249:dbl, element #13=w248:dbl)  [unwired: 13 in]
                n126 = call "管理机电流判断.vi"("数值"=w246) -> ("s? t:f"=w245:dbl)
                n127 = Bundle By Name(cluster=w261, "电池组电压"=w247, "电池组电流"=w245, "电池组温度"=w258, "母线电压"=w257, "负载电流"=w256, "母线正对地电压"=w255, "母线负对地电压"=w254, "母线正对地电阻"=w253, "母线负对地电阻"=w252, "母线对地交流电压"=w251, "主机交流输入电压A相"=w250, "主机交流输入电压B相"=w249, "主机交流输入电压C相"=w248) -> (→"管理机遥测":T4)
              }
            }
          }
          frame #1 {
            # "OPC采集"
            n128 = stacked-sequence {
              tunnel: [_ _ _ _ w335] -> w262
              frame #0 {
                # "IP10采集"
                n129 = global read "global-opc.vi" "IP10"() -> (w282:T19)
                n130 = Unbundle By Name(w282) -> ("toHMI模拟中压合闸—按钮"=w263:bool, "toHMI正常运行"=w279:bool, "toHMI异常跳闸"=w278:bool, "toHMI远程"=w277:bool, "toHMI负极柜故障报警"=w276:bool, "toHMI正极柜故障报警"=w275:bool, "toHMI馈线柜故障报警"=w274:bool, "toHMI上网柜故障报警"=w273:bool, "toHMI整流柜跳闸"=w272:bool, "toHMI整流柜合闸—状态"=w271:bool, "toHMI压敏快熔故障"=w270:bool, "toHMI整流柜故障报警"=w269:bool, "直流电流输出"=w268:u32, "直流220V电压输出"=w267:u32, "380电压输入"=w266:u32, "toHMI本地"=w264:bool)
                n131 = Bundle("直流电流输出"=w268, "直流220V电压输出"=w267, "380电压输入"=w266) -> (w265:T30)  [unwired: 1 in]
                n132 = local read "PLC-整流器柜遥信"() -> (w281:T7)
                n133 = Bundle By Name(cluster=w281, "模拟中压合闸"=w263, "正常运行"=w279, "异常跳闸"=w278, "远方"=w277, "负极柜故障"=w276, "正极柜故障"=w275, "馈线柜故障"=w274, "接触网隔离开关柜故障"=w273, "整流柜跳闸"=w272, "整流柜合闸"=w271, "压敏快熔故障"=w270, "整流柜故障"=w269, "本地"=w264) -> (w280:T7)
                n134 = local write "PLC-整流器柜遥测"(w265) -> ()
                n135 = local write "PLC-整流器柜遥信"(w280) -> ()
              }
              frame #1 {
                # "IP20采集"
                n136 = global read "global-opc.vi" "IP20"() -> (w297:T20)
                n137 = Unbundle By Name(w297) -> ("toHMI正常运行"=w294:bool, "toHMI设备准备好"=w293:bool, "toHMI设备异常"=w292:bool, "toHMI刀开关合—状态"=w291:bool, "toHMI刀开关分—状态"=w290:bool, "toHMI刀开关合按钮"=w289:bool, "toHMI刀开关分按钮"=w288:bool, "toHMI复位按钮"=w287:bool, "toHMI远程"=w286:bool, "toHMI本地"=w285:bool, "toHMI刀闸合—动作"=w284:bool, "toHMI刀闸分—动作"=w283:bool)
                n138 = local read "PLC-直流进线柜遥信"() -> (w296:T9)
                n139 = Bundle By Name(cluster=w296, "正常运行"=w294, "设备准备好"=w293, "设备异常"=w292, "刀开关合闸完成"=w291, "刀开关分闸完成"=w290, "刀开关合闸"=w289, "刀开关分闸"=w288, "复位"=w287, "远方"=w286, "本地"=w285, "刀开关合闸进行中"=w284, "刀开关分闸进行中"=w283) -> (w295:T9)
                n140 = local write "PLC-直流进线柜遥信"(w295) -> ()
              }
              frame #2 {
                # "IP30采集"
                n141 = global read "global-opc.vi" "IP30"() -> (w298:T21)
                n142 = stacked-sequence {
                  tunnel: w298 -> [_ w316]
                  frame #0 {
                  }
                  frame #1 {
                    n143 = Unbundle By Name(w316) -> ("toHMI正常运行"=w313:bool, "toHMI设备准备好"=w312:bool, "toHMI设备异常"=w311:bool, "toHMI高断合—状态"=w310:bool, "toHMI高断分—状态"=w309:bool, "toHMI继保故障信号"=w308:bool, "toHMI远方"=w307:bool, "toHMI本地"=w306:bool, "toHMI旁路合闸—按钮"=w305:bool, "toHMI旁路分闸—按钮"=w304:bool, "toHMI允许高断合闸—状态"=w303:bool, "toHMI旁路合分闸—状态"=w302:bool, "1500V电压输出"=w301:u32)
                    n144 = local read "PLC-直流馈线柜遥信"() -> (w315:T11)
                    n145 = Bundle By Name(cluster=cluster{"DC1500V电压输出":dbl} {"DC1500V电压输出"=0.0} ("PLC-直流馈线柜遥测"), "DC1500V电压输出"=w301) -> (w300:cluster{"DC1500V电压输出":dbl})
                    n146 = Bundle By Name(cluster=w315, "正常运行"=w313, "设备准备好"=w312, "设备异常"=w311, "高断合闸完成"=w310, "高断分闸完成"=w309, "继保故障信号"=w308, "远方"=w307, "本地"=w306, "旁路合闸"=w305, "旁路分闸"=w304, "允许高断合闸"=w303, "旁路合闸完成"=w302) -> (w314:T11)
                    n147 = local write "PLC-直流馈线柜遥信"(w314) -> ()
                    n148 = local write "PLC-直流馈线柜遥测"(w300) -> ()
                  }
                }
              }
              frame #3 {
                # "IP40采集"
                n149 = global read "global-opc.vi" "IP40"() -> (w334:T22)
                n150 = Unbundle By Name(w334) -> ("toHMI正常运行"=w331:bool, "toHMI设备准备好"=w330:bool, "toHMI设备异常"=w329:bool, "toHMI刀开关分—状态"=w318:bool, "toHMI刀开关合—状态"=w317:bool, "toHMI框架电流故障"=w328:bool, "toHMI框架电压故障"=w327:bool, "toHMII段电压故障"=w326:bool, "toHMIII段电压故障"=w325:bool, "toHMI装置故障"=w324:bool, "toHMIMCB故障"=w323:bool, "toHMI刀开关合—完成"=w322:bool, "toHMI复位按钮"=w321:bool, "toHMI远程"=w320:bool, "toHMI本地"=w319:bool)
                n151 = local read "PLC-负极柜遥信"() -> (w333:T13)
                n152 = Bundle By Name(cluster=w333, "正常运行"=w331, "设备准备好"=w330, "设备异常"=w329, "刀开关分闸完成"=w318, "刀开关合闸完成"=w317, "框架电流故障"=w328, "框架电压故障"=w327, "I段电压故障"=w326, "II段电压故障"=w325, "装置故障"=w324, "MCB故障"=w323, "刀开关合闸进行中"=w322, "复位"=w321, "远方"=w320, "本地"=w319) -> (w332:T13)
                n153 = local write "PLC-负极柜遥信"(w332) -> ()
              }
              frame #4 {
                # "IP50采集"
                n154 = global read "global-opc.vi" "IP50"() -> (w349:T23)
                n155 = Unbundle By Name(w349) -> ("toHMI刀开关合—状态"=w347:bool, "toHMI刀开关分—状态"=w346:bool, "toHMI刀开关合按钮"=w345:bool, "toHMI刀开关分按钮"=w344:bool, "toHMI远程"=w343:bool, "toHMI本地"=w342:bool, "toHMI正常运行"=w341:bool, "toHMI设备准备好"=w340:bool, "toHMI设备异常"=w339:bool, "toHMI刀闸合—动作"=w338:bool, "toHMI刀闸分—动作"=w337:bool, "toHMI接触轨有压"=w336:bool)
                n156 = local read "PLC-接触网隔离开关柜遥信"() -> (w348:T14)
                n157 = Bundle By Name(cluster=w348, "刀开关合闸完成"=w347, "刀开关分闸完成"=w346, "刀开关合闸"=w345, "刀开关分闸"=w344, "远方"=w343, "本地"=w342, "正常运行"=w341, "设备准备好"=w340, "设备异常"=w339, "刀开关合闸进行中"=w338, "刀开关分闸进行中"=w337, "接触轨有压"=w336) -> (w335:T14)
                n158 = local write "PLC-接触网隔离开关柜遥信"(w335) -> ()
              }
            }
          }
        }
        n159 = case shown="真" w190 {
          tunnel: w189 -> [_ w350]
          frame False {
          }
          frame True {
            n160 = call-poly <userlib>:"Enqueue Message.vi"("Priority Message? (F)"=TRUE, "Message"="Exit", "Message Queue"=w350) -> ()  [unwired: 7 in, 2 out]
          }
        }
        n161 = flat-sequence {
          tunnel: w188 -> [_]
          frame #0 {
            n162 = Wait (ms)(milliseconds to wait=u32 10 ("等待时间（毫秒）")) -> ()  [unwired: 1 out]
          }
        }
      }
      event "PLC-整流器柜遥控.模拟中压合闸控制", "PLC-直流进线柜遥控.刀开关合闸控制", "PLC-直流进线柜遥控.刀开关分闸控制", "PLC-直流进线柜遥控.故障复位控制", "PLC-直流馈线柜遥控.高断储能控制", "PLC-直流馈线柜遥控.旁路合闸控制", "PLC-直流馈线柜遥控.旁路分闸控制", "PLC-接触网隔离开关柜遥控.刀开关合闸控制", "PLC-接触网隔离开关柜遥控.刀开关分闸控制", "PLC-负极柜遥信遥控.模拟框架电流故障控制", "PLC-负极柜遥信遥控.模拟框架电压故障控制", "PLC-负极柜遥信遥控.模拟I段电压故障", "PLC-负极柜遥信遥控.模拟II段电压故障", "PLC-负极柜遥信遥控.故障复位控制": Value Change {
        n163 = event-data() -> ("CtlRef"=w363:refnum<vi>, "NewVal"=w354:bool)  [unwired: 1 in]
        n164 = global read "远程本地T.vi" "远程本地"() -> (w361:T31)
        n165 = property class="Bool (严格)"(reference=w363) -> (reference out=w355:refnum<vi>, "Caption.Text"=w362:string)  [unwired: 1 in, 1 out]
        n166 = Unbundle By Name(w361) -> ("整流柜远程/本地"=w360:enum16{"零位", "本地", "远方"}, "进线柜远程/本地"=w359:enum16{"零位", "本地", "远方"}, "馈线柜远程/本地"=w358:enum16{"零位", "本地", "远方"}, "负极柜远程/本地"=w357:enum16{"零位", "本地", "远方"}, "上网柜远程/本地"=w356:enum16{"零位", "本地", "远方"})
        n167 = case shown="\"上网柜刀合\"" w362 {
          tunnel: w354 -> [_ w370 w378 w386 w394 w402 w410 w419 w428 w436 w444 w452 w460 w473 w481]
          tunnel: w360 -> [_ w369 _ _ _ _ _ _ _ _ _ _ _ _ _]
          tunnel: w359 -> [_ _ w377 w385 w393 _ _ _ _ _ _ _ _ _ _]
          tunnel: w358 -> [_ _ _ _ _ w401 w409 w418 _ _ _ _ _ _ _]
          tunnel: w357 -> [_ _ _ _ _ _ _ _ w427 w435 w443 w451 w459 _ _]
          tunnel: w356 -> [_ _ _ _ _ _ _ _ _ _ _ _ _ w472 w480]
          tunnel: w355 -> [_ w368 w376 w384 w392 w400 w408 w417 w426 w434 w442 w450 w458 w471 w479]
          tunnel: [_ "整流柜远方>模拟中亚合闸" ("字符串") "进线柜远方>刀开关合闸" ("字符串") "进线柜远方>刀开关分闸" ("字符串") "进线柜远方>复位" ("字符串") "馈线柜远方>高断储能控制" ("字符串") "馈线柜远方>旁路合闸" ("字符串") "馈线柜远方>旁路分闸" ("字符串") "负极柜远方>模拟框架电流故障" ("字符串") "负极柜远方>模拟框架电压故障" ("字符串") "负极柜远方>模拟I段电压故障" ("字符串") "负极柜远方>模拟II段电压故障" ("字符串") "负极柜远方>复位" ("字符串") "上网柜远方>刀开关合闸" ("字符串") "上网柜远方>刀开关分闸" ("字符串")] -> w353
          frame "假", Default {
          }
          frame "整流柜中压合" {
            n168 = case shown="\"远方\"" w369 {
              tunnel: w370 -> [_ _ w374]
              tunnel: w368 -> [_ w371 _]
              frame "零位", Default {
              }
              frame "本地" {
                n169 = property class="Bool (严格)"(reference=w371, "Value"=FALSE ("值")) -> ()  [unwired: 1 in, 2 out]
                n170 = One Button Dialog(message="该权限在本地，不可投" ("消息")) -> ()  [unwired: 1 in, 1 out]
              }
              frame "远方" {
                n171 = shared-variable "我的电脑\\PLC1200.lvlib\\10fromHMI模拟中压合闸"(w374) -> ()  [unwired: 1 in, 1 out]
              }
            }
          }
          frame "进线柜刀合" {
            n172 = case shown="\"远方\"" w377 {
              tunnel: w378 -> [_ _ w382]
              tunnel: w376 -> [_ w379 _]
              frame "零位", Default {
              }
              frame "本地" {
                n173 = property class="Bool (严格)"(reference=w379, "Value"=FALSE ("值")) -> ()  [unwired: 1 in, 2 out]
                n174 = One Button Dialog(message="该权限在本地，不可投" ("消息")) -> ()  [unwired: 1 in, 1 out]
              }
              frame "远方" {
                n175 = shared-variable "我的电脑\\PLC1200.lvlib\\20fromHMI刀闸合—控制"(w382) -> ()  [unwired: 1 in, 1 out]
              }
            }
          }
          frame "进线柜刀分" {
            n176 = case shown="\"远方\"" w385 {
              tunnel: w386 -> [_ _ w390]
              tunnel: w384 -> [_ w387 _]
              frame "零位", Default {
              }
              frame "本地" {
                n177 = property class="Bool (严格)"(reference=w387, "Value"=FALSE ("值")) -> ()  [unwired: 1 in, 2 out]
                n178 = One Button Dialog(message="该权限在本地，不可投" ("消息")) -> ()  [unwired: 1 in, 1 out]
              }
              frame "远方" {
                n179 = shared-variable "我的电脑\\PLC1200.lvlib\\20fromHMI刀闸分—控制"(w390) -> ()  [unwired: 1 in, 1 out]
              }
            }
          }
          frame "进线柜复位" {
            n180 = case shown="\"远方\"" w393 {
              tunnel: w394 -> [_ _ w398]
              tunnel: w392 -> [_ w395 _]
              frame "零位", Default {
              }
              frame "本地" {
                n181 = property class="Bool (严格)"(reference=w395, "Value"=FALSE ("值")) -> ()  [unwired: 1 in, 2 out]
                n182 = One Button Dialog(message="该权限在本地，不可投" ("消息")) -> ()  [unwired: 1 in, 1 out]
              }
              frame "远方" {
                n183 = shared-variable "我的电脑\\PLC1200.lvlib\\20fromHMI故障复位"(w398) -> ()  [unwired: 1 in, 1 out]
              }
            }
          }
          frame "高断储能控制" {
            n184 = case shown="\"远方\"" w401 {
              tunnel: w402 -> [_ _ w406]
              tunnel: w400 -> [_ w403 _]
              frame "零位", Default {
              }
              frame "本地" {
                n185 = property class="Bool (严格)"(reference=w403, "Value"=FALSE ("值")) -> ()  [unwired: 1 in, 2 out]
                n186 = One Button Dialog(message="该权限在本地，不可投" ("消息")) -> ()  [unwired: 1 in, 1 out]
              }
              frame "远方" {
                n187 = shared-variable "我的电脑\\PLC1200.lvlib\\30fromHMI高断储能—控制"(w406) -> ()  [unwired: 1 in, 1 out]
              }
            }
          }
          frame "旁路合闸控制" {
            n188 = case shown="\"远方\"" w409 {
              tunnel: w410 -> [_ _ w414]
              tunnel: w408 -> [_ w411 _]
              frame "零位", Default {
              }
              frame "本地" {
                n189 = property class="Bool (严格)"(reference=w411, "Value"=FALSE ("值")) -> ()  [unwired: 1 in, 2 out]
                n190 = One Button Dialog(message="该权限在本地，不可投" ("消息")) -> ()  [unwired: 1 in, 1 out]
              }
              frame "远方" {
                n191 = shared-variable "我的电脑\\PLC1200.lvlib\\30fromHMI旁路合闸—控制"(w414) -> ()  [unwired: 1 in, 1 out]
                n192 = Not(x=w414) -> (.not. x?=w415:bool)
                n193 = property on="旁路分闸控制" class="Bool (严格)"("Value"=w415) -> ()  [unwired: 2 in, 2 out]
              }
            }
          }
          frame "旁路分闸控制" {
            n194 = case shown="\"远方\"" w418 {
              tunnel: w419 -> [_ _ w424]
              tunnel: w417 -> [_ w420 _]
              frame "零位", Default {
              }
              frame "本地" {
                n195 = property class="Bool (严格)"(reference=w420, "Value"=FALSE ("值")) -> ()  [unwired: 1 in, 2 out]
                n196 = One Button Dialog(message="该权限在本地，不可投" ("消息")) -> ()  [unwired: 1 in, 1 out]
              }
              frame "远方" {
                n197 = shared-variable "我的电脑\\PLC1200.lvlib\\30fromHMI旁路分闸—控制"(w424) -> ()  [unwired: 1 in, 1 out]
                n198 = Not(x=w424) -> (.not. x?=w423:bool)
                n199 = property on="旁路合闸控制" class="Bool (严格)"("Value"=w423) -> ()  [unwired: 2 in, 2 out]
              }
            }
          }
          frame "模拟框架电流故障控制" {
            n200 = case shown="\"远方\"" w427 {
              tunnel: w428 -> [_ _ w432]
              tunnel: w426 -> [_ w429 _]
              frame "零位", Default {
              }
              frame "本地" {
                n201 = property class="Bool (严格)"(reference=w429, "Value"=FALSE ("值")) -> ()  [unwired: 1 in, 2 out]
                n202 = One Button Dialog(message="该权限在本地，不可投" ("消息")) -> ()  [unwired: 1 in, 1 out]
              }
              frame "远方" {
                n203 = shared-variable "我的电脑\\PLC1200.lvlib\\40fromHMI模拟框架电流故障"(w432) -> ()  [unwired: 1 in, 1 out]
              }
            }
          }
          frame "模拟框架电压故障控制" {
            n204 = case shown="\"远方\"" w435 {
              tunnel: w436 -> [_ _ w440]
              tunnel: w434 -> [_ w438 _]
              frame "零位", Default {
              }
              frame "本地" {
                n205 = property class="Bool (严格)"(reference=w438, "Value"=FALSE ("值")) -> ()  [unwired: 1 in, 2 out]
                n206 = One Button Dialog(message="该权限在本地，不可投" ("消息")) -> ()  [unwired: 1 in, 1 out]
              }
              frame "远方" {
                n207 = shared-variable "我的电脑\\PLC1200.lvlib\\40fromHMI模拟框架电压故障"(w440) -> ()  [unwired: 1 in, 1 out]
              }
            }
          }
          frame "模拟I段电压故障" {
            n208 = case shown="\"远方\"" w443 {
              tunnel: w444 -> [_ _ w448]
              tunnel: w442 -> [_ w445 _]
              frame "零位", Default {
              }
              frame "本地" {
                n209 = property class="Bool (严格)"(reference=w445, "Value"=FALSE ("值")) -> ()  [unwired: 1 in, 2 out]
                n210 = One Button Dialog(message="该权限在本地，不可投" ("消息")) -> ()  [unwired: 1 in, 1 out]
              }
              frame "远方" {
                n211 = shared-variable "我的电脑\\PLC1200.lvlib\\40fromHMI模拟I段电压故障"(w448) -> ()  [unwired: 1 in, 1 out]
              }
            }
          }
          frame "模拟II段电压故障" {
            n212 = case shown="\"远方\"" w451 {
              tunnel: w452 -> [_ _ w456]
              tunnel: w450 -> [_ w453 _]
              frame "零位", Default {
              }
              frame "本地" {
                n213 = property class="Bool (严格)"(reference=w453, "Value"=FALSE ("值")) -> ()  [unwired: 1 in, 2 out]
                n214 = One Button Dialog(message="该权限在本地，不可投" ("消息")) -> ()  [unwired: 1 in, 1 out]
              }
              frame "远方" {
                n215 = shared-variable "我的电脑\\PLC1200.lvlib\\40fromHMI模拟II段电压故障"(w456) -> ()  [unwired: 1 in, 1 out]
              }
            }
          }
          frame "负机柜复位" {
            n216 = case shown="\"远方\"" w459 {
              tunnel: w460 -> [_ _ w469]
              tunnel: w458 -> [_ w461 _]
              frame "零位", Default {
              }
              frame "本地" {
                n217 = property class="Bool (严格)"(reference=w461, "Value"=FALSE ("值")) -> ()  [unwired: 1 in, 2 out]
                n218 = One Button Dialog(message="该权限在本地，不可投" ("消息")) -> ()  [unwired: 1 in, 1 out]
              }
              frame "远方" {
                w465 = FALSE
                n219 = shared-variable "我的电脑\\PLC1200.lvlib\\40fromHMI模拟框架电流故障"(w465) -> (error out=w468:errorcluster)  [unwired: 1 in]
                n220 = shared-variable "我的电脑\\PLC1200.lvlib\\40fromHMI模拟框架电压故障"(w465, error in=w468) -> (error out=w467:errorcluster)
                n221 = shared-variable "我的电脑\\PLC1200.lvlib\\40fromHMI模拟I段电压故障"(w465, error in=w467) -> (error out=w466:errorcluster)
                n222 = shared-variable "我的电脑\\PLC1200.lvlib\\40fromHMI模拟II段电压故障"(w465, error in=w466) -> (error out=w464:errorcluster)
                n223 = shared-variable "我的电脑\\PLC1200.lvlib\\40fromHMI故障复位"(w469, error in=w464) -> ()  [unwired: 1 out]
              }
            }
          }
          frame "上网柜刀合" {
            n224 = case shown="\"远方\"" w472 {
              tunnel: w473 -> [_ _ w477]
              tunnel: w471 -> [_ w474 _]
              frame "零位", Default {
              }
              frame "本地" {
                n225 = property class="Bool (严格)"(reference=w474, "Value"=FALSE ("值")) -> ()  [unwired: 1 in, 2 out]
                n226 = One Button Dialog(message="该权限在本地，不可投" ("消息")) -> ()  [unwired: 1 in, 1 out]
              }
              frame "远方" {
                n227 = shared-variable "我的电脑\\PLC1200.lvlib\\50fromHMI刀闸合—控制"(w477) -> ()  [unwired: 1 in, 1 out]
              }
            }
          }
          frame "上网柜刀分" {
            n228 = case shown="\"远方\"" w480 {
              tunnel: w481 -> [_ _ w485]
              tunnel: w479 -> [_ w482 _]
              frame "零位", Default {
              }
              frame "本地" {
                n229 = property class="Bool (严格)"(reference=w482, "Value"=FALSE ("值")) -> ()  [unwired: 1 in, 2 out]
                n230 = One Button Dialog(message="该权限在本地，不可投" ("消息")) -> ()  [unwired: 1 in, 1 out]
              }
              frame "远方" {
                n231 = shared-variable "我的电脑\\PLC1200.lvlib\\50fromHMI刀闸分—控制"(w485) -> ()  [unwired: 1 in, 1 out]
              }
            }
          }
        }
        n232 = case shown="真" w354 {
          tunnel: w353 -> [_ w365]
          frame False {
          }
          frame True {
            n233 = call "报警更新.vi"("Message Data"=w365, "state"="动作更新") -> ()  [unwired: 10 in]
          }
        }
      }
      event "继保遥控.断路器分闸", "继保遥控.断路器合闸", "PLC-直流馈线柜遥控.断路器分闸", "PLC-直流馈线柜遥控.断路器合闸": Value Change {
        n234 = event-data() -> ("CtlRef"=w493:refnum<vi>, "NewVal"=w486:bool)  [unwired: 1 in, 3 out]
        n235 = global read "global-opc.vi" "IP30"() -> (w491:T21)
        n236 = Unbundle By Name(w491) -> ("toHMI远方"=w487:bool, "toHMI高断分—状态"=w489:bool, "toHMI高断合—状态"=w490:bool)
        n237 = property class="Bool (严格)"(reference=w493) -> (reference out=w488:refnum<vi>, "Label.Text"=w492:string)  [unwired: 1 in, 1 out]
        n238 = case shown="真" w487 {
          tunnel: w492 -> [_ w502]
          tunnel: w486 -> [_ w498]
          tunnel: w490 -> [_ w501]
          tunnel: w489 -> [_ w500]
          tunnel: w488 -> [w496 w499]
          frame False {
            n239 = property class="Bool (严格)"(reference=w496, "Value"=FALSE ("值")) -> ()  [unwired: 1 in, 2 out]
            n240 = One Button Dialog(message="该权限在本地，不可投" ("消息")) -> ()  [unwired: 1 in, 1 out]
          }
          frame True {
            n241 = case shown="真" w498 {
              tunnel: w502 -> [_ w508]
              tunnel: w501 -> [_ w507]
              tunnel: w500 -> [_ w506]
              tunnel: w499 -> [_ w505]
              frame False {
              }
              frame True {
                n242 = case shown="\"断路器分闸\", 默认" w508 {
                  tunnel: w507 -> [w509 _]
                  tunnel: w506 -> [_ w521]
                  tunnel: w505 -> [w511 w523]
                  tunnel: ["直流继保远方>高速断路器分闸" ("字符串") "直流继保远方>高速断路器合闸" ("字符串")] -> w503
                  frame "断路器分闸", Default {
                    n243 = case shown="真" w509 {
                      tunnel: w511 -> [w512 _]
                      frame False {
                        n244 = property class="Bool (严格)"(reference=w512, "Value"=FALSE ("值")) -> ()  [unwired: 1 in, 2 out]
                        n245 = One Button Dialog(message="高速断路器已分闸" ("消息")) -> ()  [unwired: 1 in, 1 out]
                      }
                      frame True {
                        n246 = call <userlib>:"Obtain Message Queue.vi"("name (unnamed)"="继保.vi") -> ("Message Queue"=w520:refnum<queue>)  [unwired: 9 in, 1 out]
                        n247 = Bundle(u16 256, TRUE) -> (w516:cluster{u16, bool})  [unwired: 1 in]
                        n248 = call-poly <userlib>:"Enqueue Message.vi"("Message Data"=w516, "Message"="遥控", "Message Queue"=w520) -> ()  [unwired: 7 in, 2 out]
                      }
                    }
                  }
                  frame "断路器合闸" {
                    n249 = case shown="真" w521 {
                      tunnel: w523 -> [w526 _]
                      frame False {
                        n250 = property class="Bool (严格)"(reference=w526, "Value"=FALSE ("值")) -> ()  [unwired: 1 in, 2 out]
                        n251 = One Button Dialog(message="高速断路器已合闸" ("消息")) -> ()  [unwired: 1 in, 1 out]
                      }
                      frame True {
                        n252 = call <userlib>:"Obtain Message Queue.vi"("name (unnamed)"="继保.vi") -> ("Message Queue"=w532:refnum<queue>)  [unwired: 9 in, 1 out]
                        n253 = Bundle(u16 257, TRUE) -> (w528:cluster{u16, bool})  [unwired: 1 in]
                        n254 = call-poly <userlib>:"Enqueue Message.vi"("Message Data"=w528, "Message"="遥控", "Message Queue"=w532) -> ()  [unwired: 7 in, 2 out]
                      }
                    }
                  }
                }
                n255 = call "报警更新.vi"("Message Data"=w503, "state"="动作更新") -> ()  [unwired: 10 in]
              }
            }
          }
        }
      }
      event Panel Close? {
        # "Send the 'Confirm Quit' message if the user closes the panel of the VI. Discard the event so the 'Confirm Quit' message has a chance to run."
        n256 = event-data() -> ()  [unwired: 1 in, 1 out]
        n257 = call-poly <userlib>:"Enqueue Message.vi"("Priority Message? (F)"=TRUE, "Message"="Confirm Quit", "Message Queue"=w537) -> ("error out"=w536:errorcluster, "dup Message Queue"=w535:refnum<queue>)  [unwired: 7 in]
        n258 = event-data("Discard?"=TRUE) -> ()  [unwired: 1 in, 1 out]
      }
      event Application Instance Close {
        # "#CodeRecommended - When a project closes, all VIs within that project are aborted and leave memory. However, any code placed in this event frame is guaranteed to run to completion, so add any cleanup code that absolutely must happen here."
        n259 = event-data() -> ()  [unwired: 1 in, 1 out]
      }
      event User Event {
        # "The Message Handling Loop processed an \"Exit\" message, which fired this event to stop the Event Handling Loop."
        n260 = event-data() -> ()  [unwired: 1 in, 1 out]
      }
      event "Exit": Value Change {
        # "Exit all of the program,and do not change the Box"
        n261 = event-data() -> ()  [unwired: 1 in, 1 out]
        n262 = call-poly <userlib>:"Enqueue Message.vi"("Priority Message? (F)"=TRUE, "Message"="Confirm Quit", "Message Queue"=w546) -> ("error out"=w544:errorcluster, "dup Message Queue"=w545:refnum<queue>)  [unwired: 7 in]
      }
      event "切换界面": Shortcut Menu Selection (User) {
        n263 = event-data() -> ("ItemTag"=w548:string)  [unwired: 1 in, 1 out]
        n264 = case shown="\"管理机监控\", 默认" w548 {
          tunnel: [enum32{"继保信号", "管理机信号", "柜体信号"}."管理机信号" ("选项卡控件") enum32{"继保信号", "管理机信号", "柜体信号"}."继保信号" ("选项卡控件") enum32{"继保信号", "管理机信号", "柜体信号"}."柜体信号" ("选项卡控件")] -> w547
          frame "管理机监控", Default {
          }
          frame "继保监控" {
          }
          frame "柜体监控" {
          }
        }
        n265 = local write "选项卡控件"(w547) -> ()
      }
      event "切换界面": Value Change {
        n266 = event-data() -> ("NewVal"=w553:bool)  [unwired: 1 in, 5 out]
        n267 = case shown="真" w553 {
          frame False {
          }
          frame True {
            n268 = local read "选项卡控件"() -> (w556:enum32{"继保信号", "管理机信号", "柜体信号"})
            n269 = Increment(x=w556) -> (x+1=w558:enum32{"继保信号", "管理机信号", "柜体信号"})
            n270 = Quotient & Remainder(x=w558, y=3) -> (x-y*floor(x/y)=w555:u32)  [unwired: 1 out]
            n271 = local write "选项卡控件"(w555) -> ()
          }
        }
      }
      event "直流屏-遥信", "直流屏-遥测": Value Change {
        n272 = event-data() -> ("CtlRef"=w564:refnum<vi>)  [unwired: 1 in]
        n273 = property class="Bool (严格)"(reference=w564) -> (reference out=w559:refnum<vi>, "Label.Text"=w563:string, "Value"=w562:bool)  [unwired: 1 in, 1 out]
        n274 = Variant To Data(type=FALSE, Variant=w562) -> (data=w560:bool)  [unwired: 1 in, 1 out]
        n275 = case shown="真" w560 {
          tunnel: w563 -> [_ w568]
          tunnel: w559 -> [_ w567]
          frame False {
          }
          frame True {
            n276 = case shown="\"直流屏-遥信\"" w568 {
              tunnel: w567 -> [_ _]
              tunnel: [enum32{"管遥信", "管遥测"}."管遥测" ("管理机选项卡") enum32{"管遥信", "管遥测"}."管遥信" ("管理机选项卡")] -> w566
              frame "直流屏-遥测", Default {
              }
              frame "直流屏-遥信" {
              }
            }
            n277 = local write "管理机选项卡"(w566) -> ()
          }
        }
      }
    }
    n278 = call <userlib>:"Error Handler - Event Handling Loop.vi"("error in (no error)"=w184, "Message Queue"=w182) -> ("dup error in"=w181:errorcluster)  [unwired: 8 in, 1 out]
  }
  n279 = Unregister For Events(event registration refnum=w16, error in=w15) -> (error out=w17:errorcluster)
  n280 = Merge Errors(w17, w21) -> (w19:errorcluster)
  n281 = call <userlib>:"Destroy User Event - Stop.vi"("error in (no error)"=w19, "User Event - Stop"=w18) -> ()  [unwired: 9 in, 1 out]
